vi "Get Graph.vi"(11 "Base Graph in":refnum<class "Base Graph.lvclass">) -> (2 "Graph":refnum<vi>, 3 "Base Graph out":refnum<class "Base Graph.lvclass">)   [LabVIEW 2023, in "Base Graph.lvclass"]
uses:
  Base Graph.lvclass
  Base Graph.lvclass/Base Graph.ctl
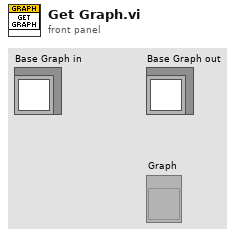
[diagram p1: front panel]
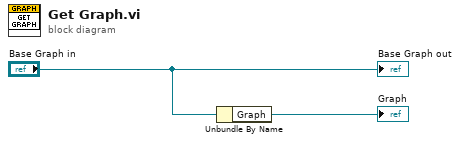
[diagram p0: block diagram]
diagram:
  n1 = Unbundle By Name("Base Graph in") -> ("Graph"=→"Graph":refnum<vi>)
  "Base Graph out" <- "Base Graph in"
